vi "Write Rounding Size.vi"(8 "error in (no error)":errorcluster, 10 "Rounding Size":cluster{"Width":i16, "Height":i16}, 11 "Rectangle in":refnum<class "Rectangle.lvclass">) -> (0 "error out":errorcluster, 3 "Rectangle out":refnum<class "Rectangle.lvclass">)   [LabVIEW 2017, in "LV Image Editor Framework.lvlib" / "Rectangle.lvclass"]
uses:
  <vilib>/LIEF/Forms/Rectangle/Rectangle.lvclass
  <vilib>/LIEF/Forms/Rectangle/Rectangle.lvclass/Rectangle.ctl
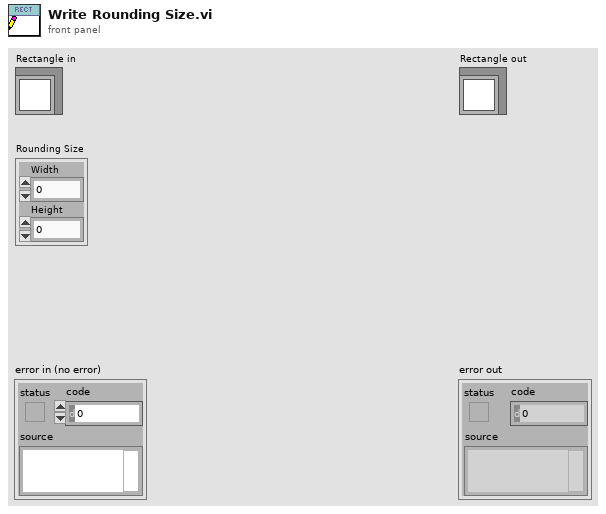
[diagram p1: front panel]
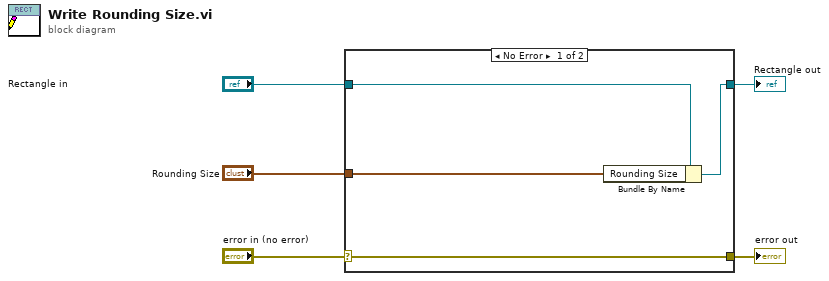
[diagram p0: block diagram]
diagram:
  n1 = case shown="No Error" "error in (no error)" {
    selector: "error in (no error)" -> [w9 w10]
    tunnel: [w9 w10] -> w4
    tunnel: [w7 w11] -> w2
    tunnel: "Rectangle in" -> [w8 w11]
    tunnel: "Rounding Size" -> [w6 _]
    frame No Error {
      n2 = Bundle By Name(cluster=w8, "Rounding Size"=w6) -> (w7:refnum<class "Rectangle.lvclass">)
    }
    frame Error {
    }
  }
  "error out" <- w4
  "Rectangle out" <- w2
